vi "Keithley2400_SR830_LakeShore336_4Probe_Resistance_Measurement.vi"() -> ()   [LabVIEW 2018]
uses:
  <instrlib>/Lake Shore 336/Public/Data/Sensor Data (Single Reading).vi
  <instrlib>/Stanford Research 830/Public/Data/Read (All Parameters).vi
  <instrlib>/Keithley 24XX/Public/Data/Read (Single Point).vi
  <instrlib>/Keithley 24XX/Keithley 24XX.lvlib
  <instrlib>/Stanford Research 830/Stanford Research 830.lvlib
  <instrlib>/Lake Shore 336/Lake Shore 336.lvlib
panel:
  out "Gate\nVoltage":sgl
  out "Status":sgl
  out "Leakage \nCurrent":sgl
  in  "Temp Vs Time":enum32{"XY Graph", "Waveform (Time)"}(tab)
  out "Temp vs Time : XYGraph":cluster{"Y":dbl[], "Y":dbl[]}[](graph)
  out "Temp vs Time : TimeGraph":cluster{i32, "Sensor Data":dbl}[](graph)
  in  "Data Source (0:Kelvin)":u16(ring) items=["Kelvin", "Celsius", "Sensor Units"]
  in  "Input (0:A)":u16(ring) items=["A", "B", "C", "D"]
  in  "Serial Configuration 2":T1={"Baud Rate"=57600, "Parity"=1, "Data Bits"=7, "Stop Bits"=10, "Flow Control"=0} {"Flow Control" items=["None", "XON/XOFF", "RTS/CTS", "XON/XOFF & RTS/CTS", "DTR/DSR", "XON/XOFF & DTR/DSR"]; "Stop Bits" items=["1.0"=10, "1.5"=15, "2.0"=20]; "Data Bits" items=["7"=7, "8"=8]; "Parity" items=["None", "Odd", "Even", "Mark", "Space"]; "Baud Rate" items=["300"=300, "600"=600, "1200"=1200, "2400"=2400, "4800"=4800, "9600"=9600, "19200"=19200, "38400"=38400, "57600"=57600]}
  in  "LakeShore 336 esource name":refnum<visa-resource-name>="GPIB0::12::INSTR"
  out "dup path":path
  in  "<File Name>.txt (Don't add extension)":string
  in  "Data Save Path:":path=path "C:/Users/labpc/Documents/ProbeStation Users Data"
  in  "I_leak vs Vg":enum32{"XY Graph", "Waveform (Time)"}(tab)
  out "I_leak vs Vg : XYGraph":cluster{"Y":dbl[], "Y":dbl[]}[](graph)
  out "I_leak vs Vg : TimeGraph":cluster{dbl, "Current":sgl}[](graph)
  in  "Gate Voltage\nInitial (V)":dbl
  out "Gate Voltage\nTraversal Direction":enum16{"Upward", "Downward"}(ring)
  in  "Series Resistance \n(Apparatus Constant)":dbl=10000000.0
  in  "stop":bool
  out "Max/Min(-) \nGate Voltage (V)":dbl=80.0
  in  "Gate Voltage \nStep Size (V)":dbl=0.1
  in  "High Gate \nVoltage (V)":dbl
  in  "Low Gate \nVoltage (V)":dbl
  out "Compliance\n Level (A)":dbl=0.1
  in  "Theta vs Vg":enum32{"XY Graph", "Waveform (Time)"}(tab)
  out "Theta vs Vg : XYGraph":cluster{"Y":dbl[], "Y":dbl[]}[](graph)
  out "Theta vs Vg : TimeGraph":cluster{dbl, "Theta-Value":dbl}[](graph)
  in  "R vs Vg":enum32{"XY Graph", "Waveform (Time)"}(tab)
  out "Resistance vs Vg : XYGraph":cluster{"Y":dbl[], "Y":dbl[]}[](graph)
  out "R vs Vg : TimeGraph":cluster{dbl, dbl}[](graph)
  in  "Sensitivity (Initial Value)":i16(ring)=17 items=["Auto Gain"=-1, "2 nV/fA"=0, "5 nV/fA"=1, "10 nV/fA"=2, "20 nV/fA"=3, "50 nV/fA"=4, "100 nV/fA"=5, "200 nV/fA"=6, "500 nV/fA"=7, "1 uV/pA"=8, "2 uV/pA"=9, "5 uV/pA"=10, "10 uV/pA"=11, "20 uV/pA"=12, "50 uV/pA"=13, "100 uV/pA"=14, "200 uV/pA"=15, "500 uV/pA"=16, "1 mV/nA"=17, "2 mV/nA"=18, "5 mV/nA"=19, "10 mV/nA"=20, "20 mV/nA"=21, "50 mV/nA"=22, "100 mV/nA"=23, "200 mV/nA"=24, "500 mV/mA"=25, "1 V/uA"=26]
  in  "Dynamic Reserve (-1 = Auto)":i16(ring)=-1 items=["Auto Reserve"=-1, "High Reserve"=0, "Normal"=1, "Low Noise"=2]
  in  "Input Connection (0: Single-Ended Voltage)":u16(ring)=1 items=["Single-Ended Voltage", "Differential Voltage", "1 MOhm Current Gain", "100 MOhm Current Gain"]
  out "Input Coupling (0: AC)":u16(ring) items=["AC", "DC"]
  in  "Time Constant (8: 100ms)":u16(ring)=9 items=["10 us", "30 us", "100 us", "300 us", "1 ms", "3 ms", "10 ms", "30 ms", "100 ms", "300 ms", "1 s", "3 s", "10 s", "30 s", "100 s", "300 s", "1 ks", "3 ks", "10 ks", "30 ks"]
  in  "SR830 VISA resource name":refnum<visa-resource-name>="GPIB0::10::INSTR"
  in  "Trigger Source (0: Internal)":u16(ring) items=["Internal", "External"]
  out "Manual Phase (0 Degree)":dbl
  out "Detection Harmonic Number":dbl=1.0
  out "External Reference Trigger (0: Sine Zero Crossing)":u16(ring) items=["Sine Zero Crossing", "TTL Rising Edge", "TTL Falling Edge"]
  in  "Internal Reference Frequency (1000 Hz)":dbl=17.0
  in  "Reference Source (1: Internal)":u16(ring)=1 items=["External", "Internal"]
  in  "Sine Output Amplitude (V)":dbl=1.0
  in  "Serial Configuration":T1={"Baud Rate"=9600, "Parity"=0, "Data Bits"=8, "Stop Bits"=10, "Flow Control"=0} {"Flow Control" items=["None", "XON/XOFF", "RTS/CTS", "XON/XOFF & RTS/CTS", "DTR/DSR", "XON/XOFF & DTR/DSR"]; "Stop Bits" items=["1.0"=10, "1.5"=15, "2.0"=20]; "Data Bits" items=["7"=7, "8"=8]; "Parity" items=["None", "Odd", "Even", "Mark", "Space"]; "Baud Rate" items=["300"=300, "600"=600, "1200"=1200, "2400"=2400, "4800"=4800, "9600"=9600, "19200"=19200]}
  in  "Keithley24XX VISA resource name":refnum<visa-resource-name>="GPIB0::21::INSTR" caption="Keithley 24XX VISA resource name"
  out "Interal Measurement Time":u32
  # "Lake Shore 336 Temp Contr."
  # "SR830 Lock In Amplifier"
  # "MAKE SURE THE SOURCE METER IS ON TO ENSURE NO UNINTENDED JUMPS. PROGRAM WILL KEEP SOURCE METER ON ONCE RUN."
  # "Keithley 2400 SourceMeter"
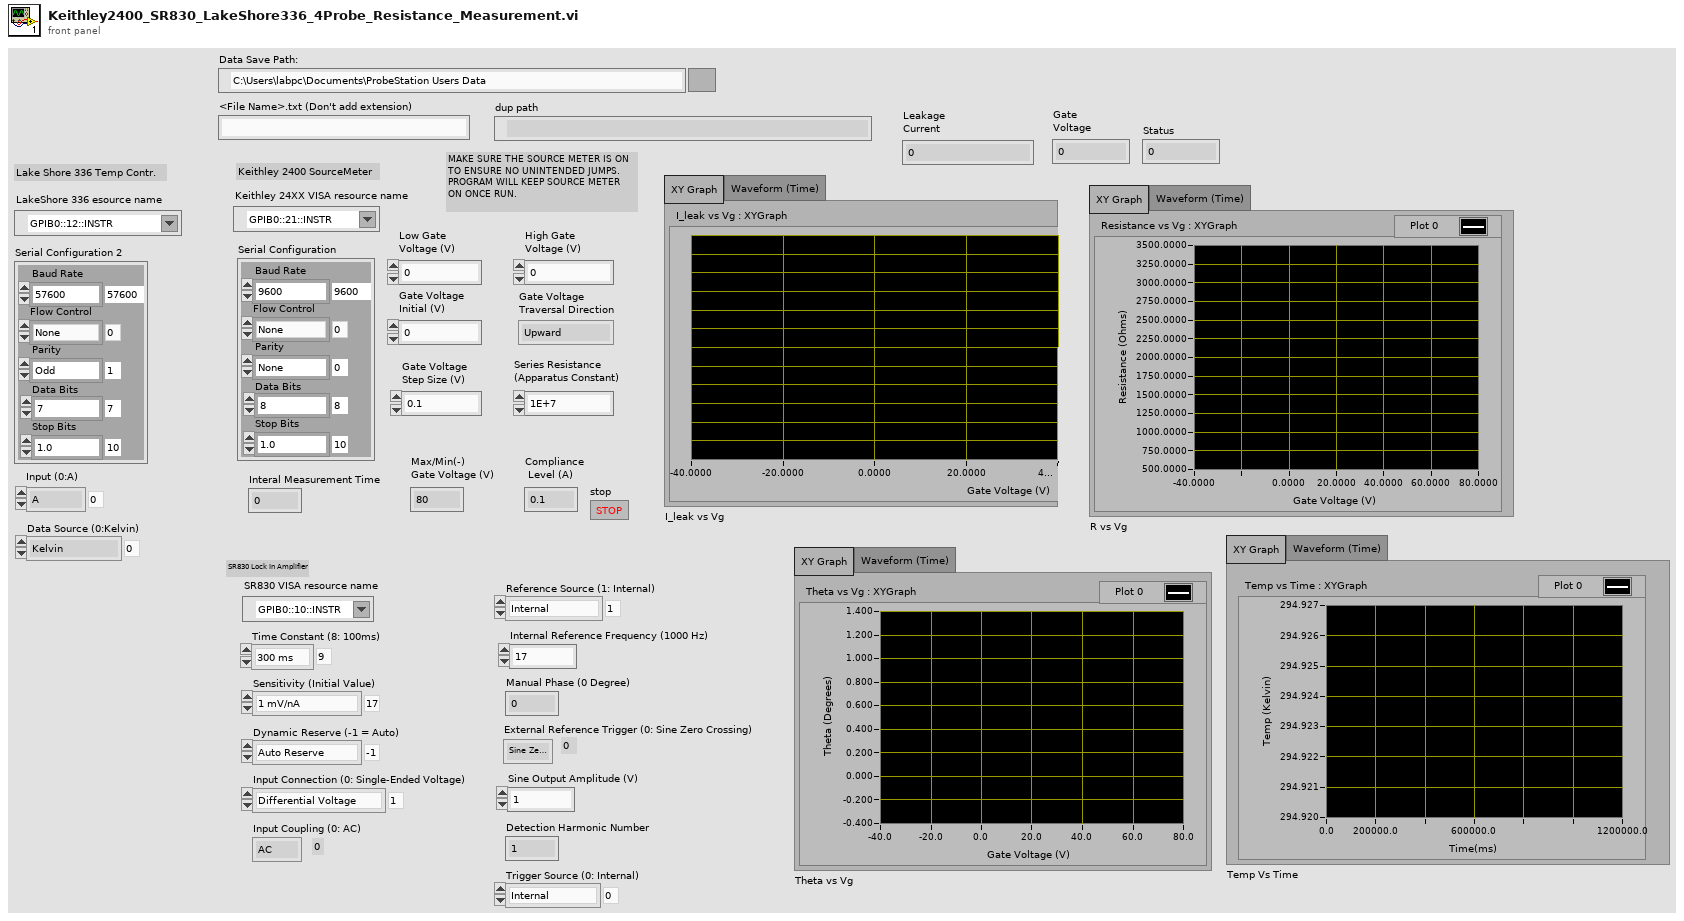
[diagram p1: front panel]
types:
  T1 = cluster{"Baud Rate":u32, "Parity":u16, "Data Bits":u16, "Stop Bits":u16, "Flow Control":u16}
  T2 = enum16{"open", "replace", "create", "open or create", "replace or create", "replace or create with confirmation"}
  T3 = cluster{"X-Value":dbl, "Y-Value":dbl, "R-Value":dbl, "Theta-Value":dbl, "Aux In 1 Value":dbl, "Aux In 2 Value":dbl, "Aux In 3 Value":dbl, "Aux In 4 Value":dbl, "Reference Frequency":dbl, "Channel 1 Display":dbl, "Channel 2 Display":dbl}
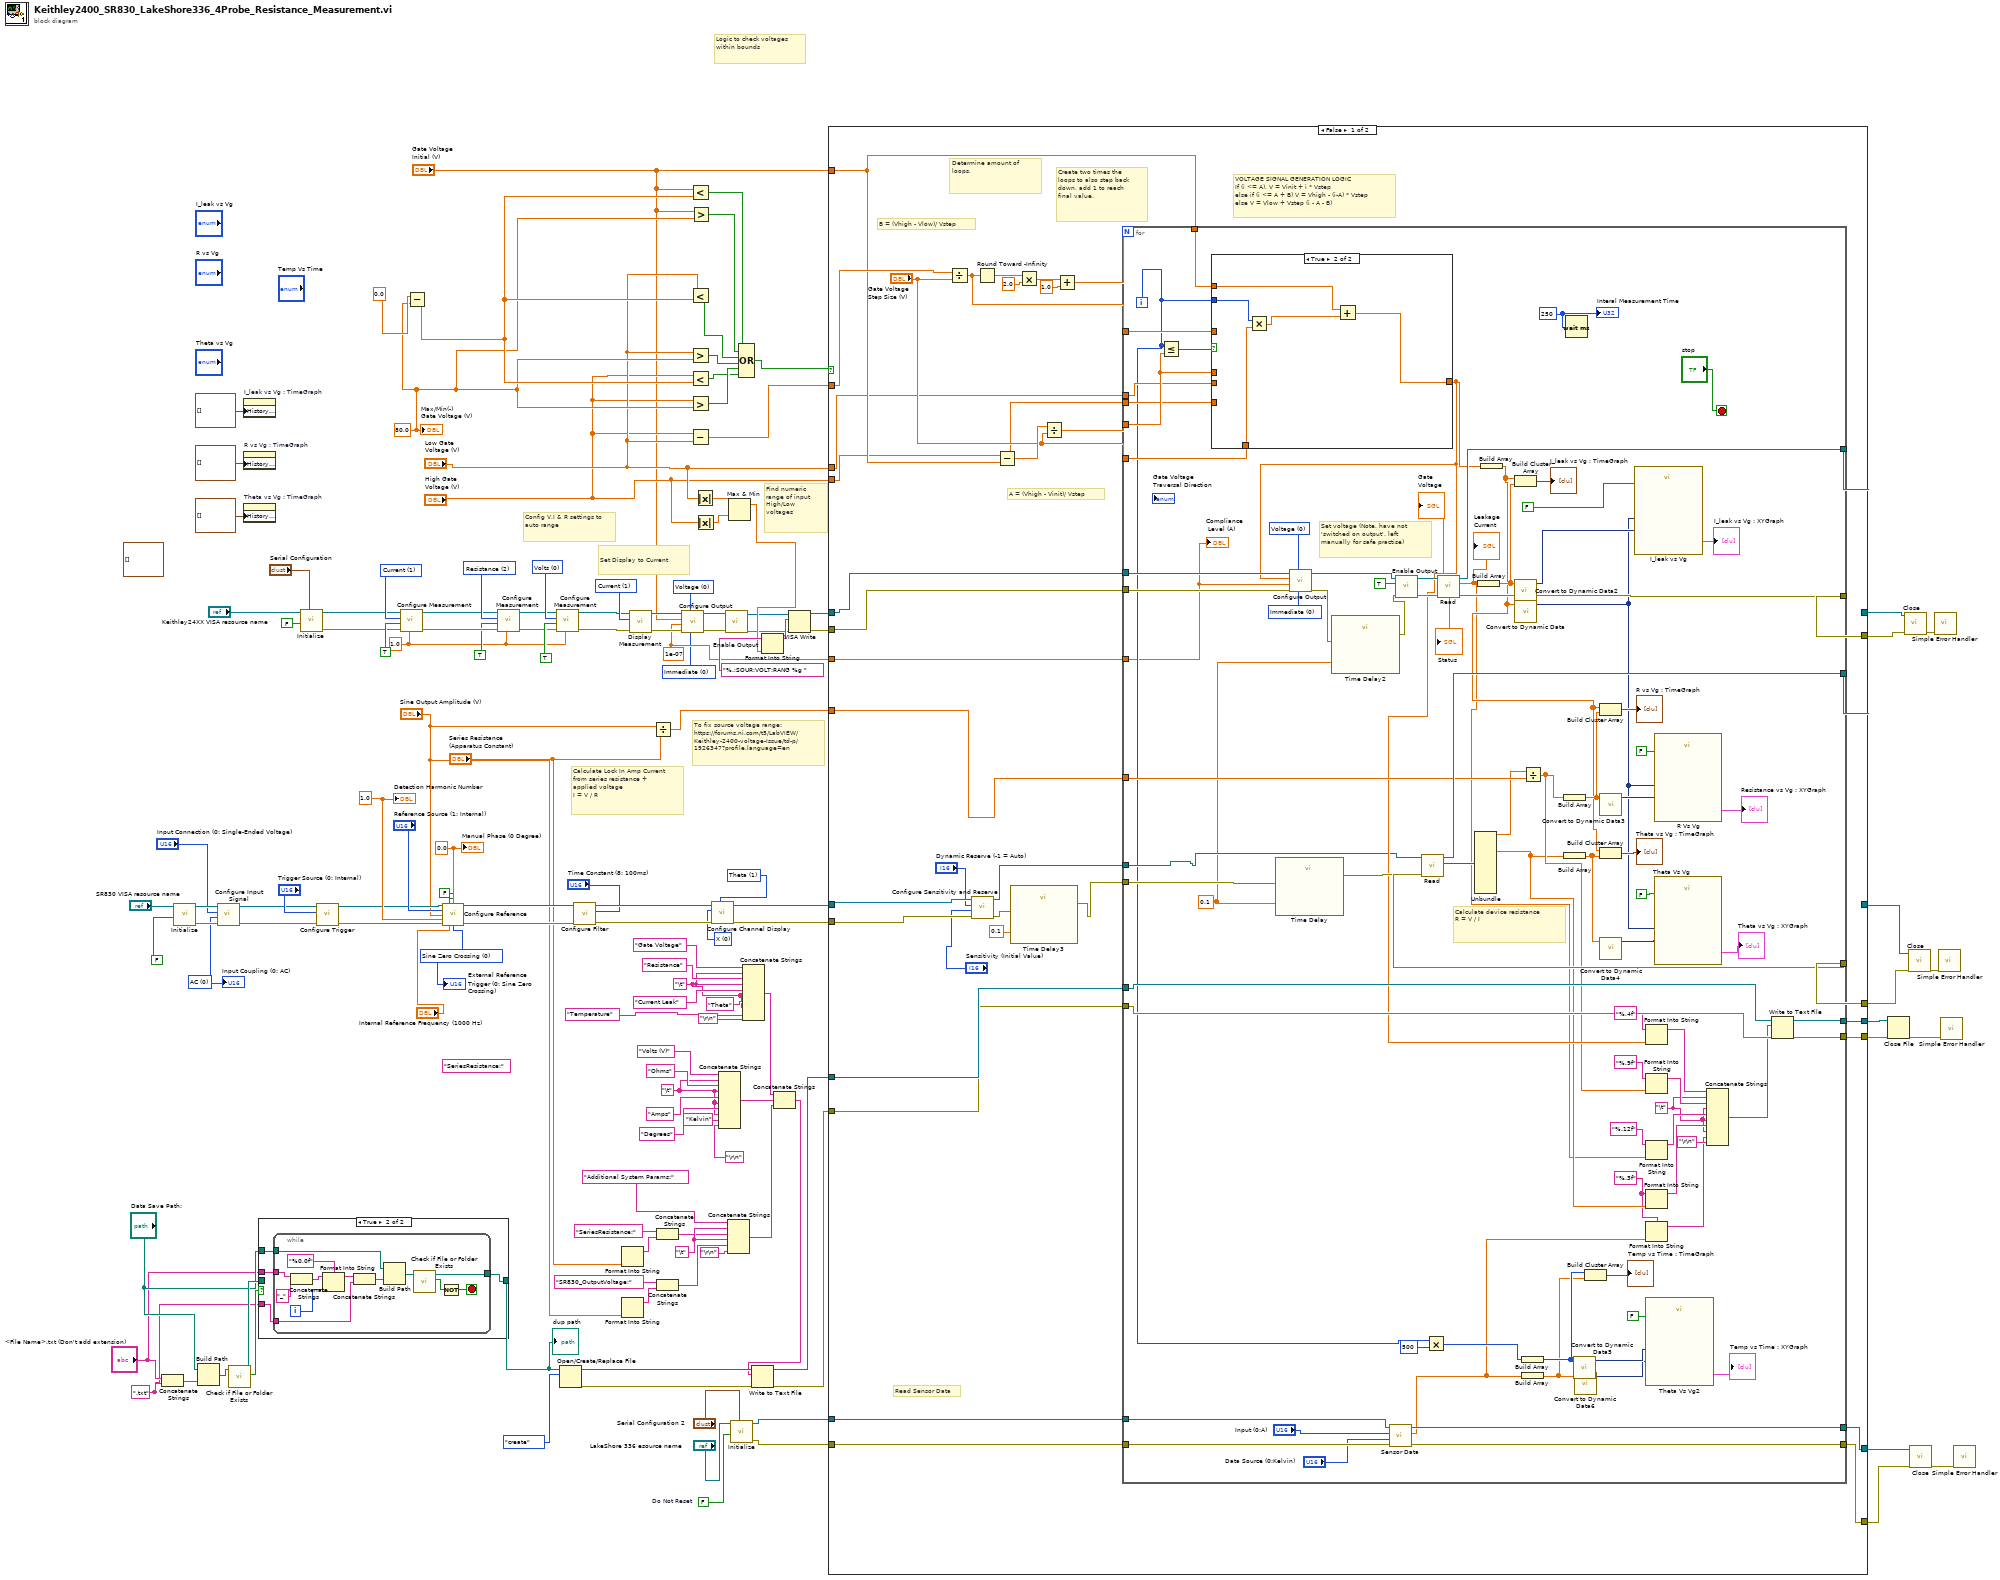
[diagram p0: block diagram]
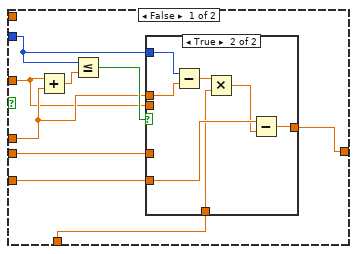
[diagram p3: hidden frame]
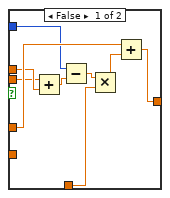
[diagram p4: hidden frame]
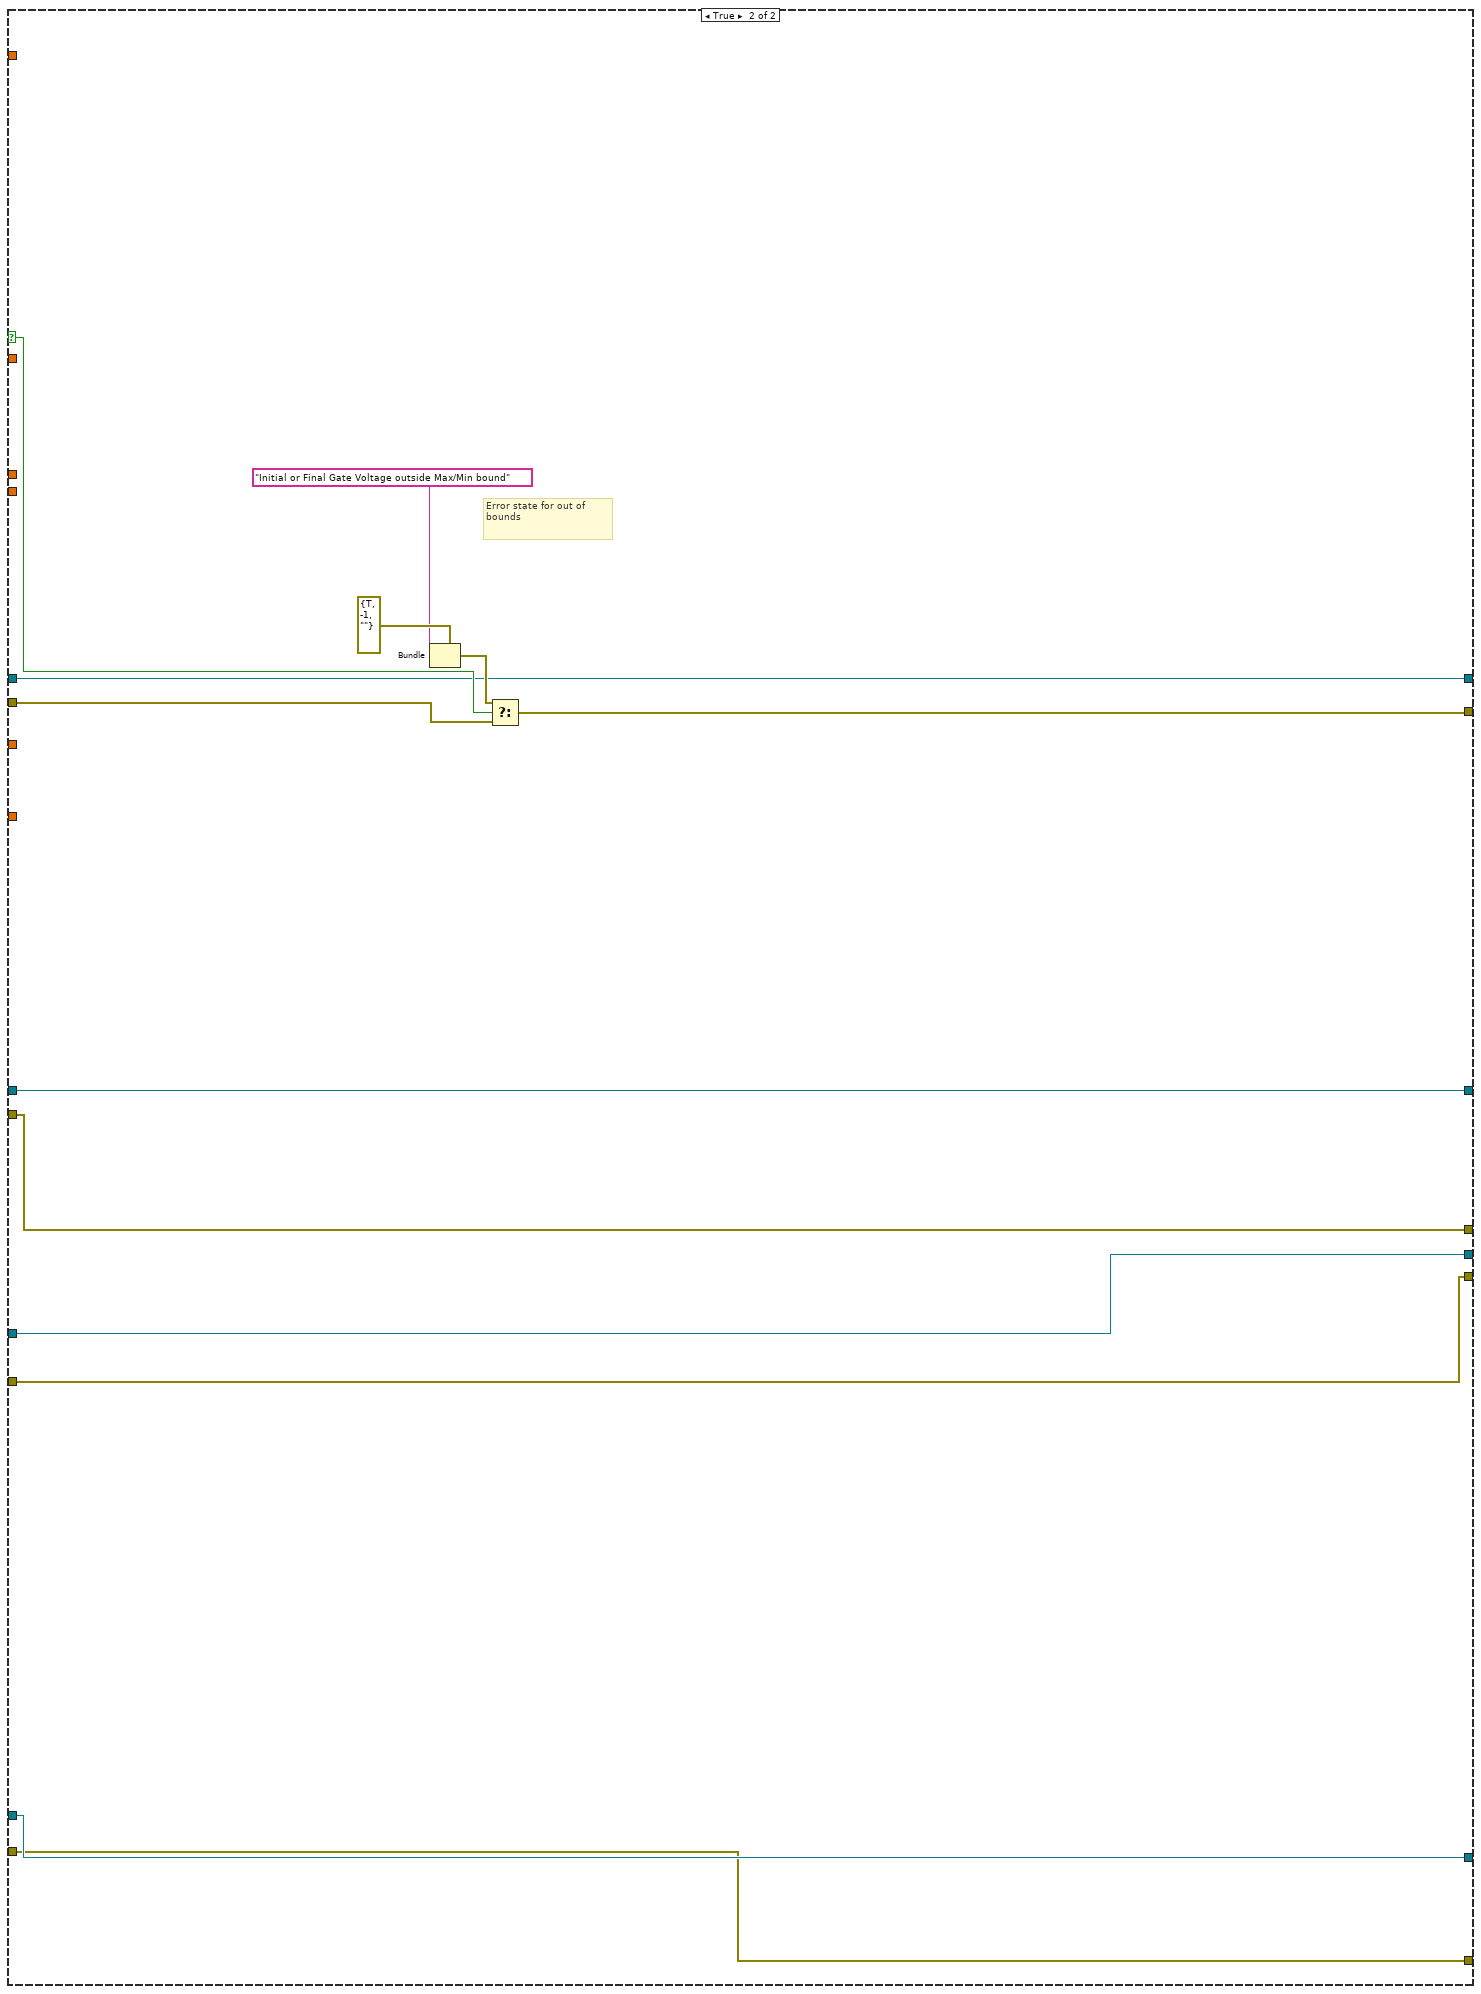
[diagram p5: hidden frame]
diagram:
  w1 = u16 0 items=["Immediate", "Triggered"] ("Output Type  (0: Immediate)")
  w2 = 1e-07 ("Compliance  Level (0.1)")
  w8 = u16 0 items=["Voltage", "Current"] ("Source Mode  (0: Voltage)")
  (unwired) cluster{dbl, "Theta-Value":dbl}[] [] ("History Data")
  w32 = FALSE  # Do Not Reset
  w38 = "\t"
  w21 = "\t"
  w23 = "\t"
  (unwired) "SeriesResistance:" ("string")
  w66 = ".txt"
  w73 = 1.0 ("Manual Range (1.0)")
  w97 = 0.0 ("Manual Phase (0 Degree)")
  w98 = 1.0 ("Detection Harmonic Number (1)")
  w99 = u16 0 items=["Sine Zero Crossing", "TTL Rising Edge", "TTL Falling Edge"] ("External Reference Trigger (0: Sine Zero Crossing)")
  w103 = u16 0 items=["AC", "DC"] ("Input Coupling (0: AC)")
  w85 = u16 0 items=["X", "R", "X Noise", "Aux In 1", "Aux In 2"] ("Channel 1 Display (0: X)")
  w113 = u16 1 items=["Y", "Theta", "Y Noise", "Aux In 3", "Aux In 4"] ("Channel 2 Display  (0: Y)")
  w118 = u16 1 items=["Voltage", "Current", "Resistance"] ("Displayed Measurement (0: Voltage)")
  w127 = u16 2 items=["Volts", "Current", "Resistance"] ("Function (0: Volts)")
  w131 = u16 1 items=["Volts", "Current", "Resistance"] ("Function (0: Volts)")
  w74 = 80.0
  w137 = u16 0 items=["Volts", "Current", "Resistance"] ("Function (0: Volts)")
  # "Find numeric range of input High/Low voltages"
  # "To fix source voltage range:\nhttps://forums.ni.com/t5/LabVIEW/Keithley-2400-voltage-Issue/td-p/1926347?profile.language=en"
  # "Logic to check voltages within bounds"
  # "Calculate Lock In Amp Current from series resistance + applied voltage\nI = V / R"
  # "Set Display to Current"
  # "Config V,I & R settings to auto range"
  n1 = Concatenate Strings("<File Name>.txt (Don't add extension)", w66) -> (w72:string)
  n2 = call <instrlib>:"Initialize.vi"("Reset (True)"=FALSE, "VISA resource name"="SR830 VISA resource name") -> ("error out"=w110:errorcluster, "VISA resource name out"=w111:refnum<visa-resource-name>)  [unwired: 8 in]
  n3 = Build Path(base path="Data Save Path:", name or relative path=w72) -> (appended path=w71:path)
  n4 = call <instrlib>:"Configure Input Signal.vi"("error in (no error)"=w110, "Input Coupling (0: AC)"=w103, "Input Connection (0: Single-Ended Voltage)"="Input Connection (0: Single-Ended Voltage)", "VISA resource name"=w111) -> ("error out"=w94:errorcluster, "VISA resource name out"=w95:refnum<visa-resource-name>)  [unwired: 6 in]
  n5 = call <vilib>:"Check if File or Folder Exists.vi"("path"=w71) -> ("file or folder exists?"=w70:bool, "dup path"=w69:path)  [unwired: 8 in, 1 out]
  n6 = property on="I_leak vs Vg : TimeGraph" class="WFChart (strict)"("History Data"=cluster{dbl, "Current":sgl}[] []) -> ()  [unwired: 2 in, 2 out]
  n7 = property on="R vs Vg : TimeGraph" class="WFChart (strict)"("History Data"=cluster{dbl, dbl}[] []) -> ()  [unwired: 2 in, 2 out]
  n8 = property on="Theta vs Vg : TimeGraph" class="WFChart (strict)"("History Data"=cluster{dbl, "Theta-Value":dbl}[] []) -> ()  [unwired: 2 in, 2 out]
  n9 = case shown="True" w70 {
    tunnel: [w139 w140] -> w63
    tunnel: w69 -> [w139 _]
    tunnel: "Data Save Path:" -> [_ w141]
    tunnel: "<File Name>.txt (Don't add extension)" -> [_ w143]
    tunnel: w66 -> [_ w142]
    frame False {
    }
    frame True {
      n10 = while {
        tunnel: w143 -> [w146]
        tunnel: w142 -> [w151]
        tunnel: w141 -> [w149]
        tunnel: [w147] -> w140
        i -> [w153]
        stop <- w155 stop-if-true
        n11 = Concatenate Strings(w146, "_" ("string")) -> (w145:string)
        n12 = Format Into String(format string="%0.0f", initial string=w145, w153) -> (resulting string=w152:string)  [unwired: 1 in, 1 out]
        n13 = Concatenate Strings(w152, w151) -> (w150:string)
        n14 = Build Path(base path=w149, name or relative path=w150) -> (appended path=w148:path)
        n15 = call <vilib>:"Check if File or Folder Exists.vi"("path"=w148) -> ("file or folder exists?"=w156:bool, "dup path"=w147:path)  [unwired: 8 in, 1 out]
        n16 = Not(x=w156) -> (.not. x?=w155:bool)
      }
    }
  }
  "dup path" <- w63
  n17 = call <instrlib>:"Initialize.vi"("Serial Configuration"="Serial Configuration", "Reset (True)"=FALSE, "VISA resource name"="Keithley24XX VISA resource name") -> ("error out"=w122:errorcluster, "VISA resource name out"=w123:refnum<visa-resource-name>)  [unwired: 7 in]
  n18 = call <instrlib>:"Configure Trigger.vi"("error in (no error)"=w94, "Trigger Source (0: Internal)"="Trigger Source (0: Internal)", "VISA resource name"=w95) -> ("error out"=w92:errorcluster, "VISA resource name out"=w93:refnum<visa-resource-name>)  [unwired: 7 in]
  n19 = call <instrlib>:"Configure Measurement.vi"("Manual Range (1.0)"=w73, "error in (no error)"=w122, "Enable Auto Range (T:Enable)"=TRUE, "Function (0: Volts)"=w131, "VISA resource name"=w123) -> ("error out"=w129:errorcluster, "VISA resource name out"=w124:refnum<visa-resource-name>)  [unwired: 5 in]
  n20 = Subtract(x=0.0, y=w74) -> (x-y=w79:dbl)
  n21 = call <instrlib>:"Configure Reference.vi"("VISA resource name"=w93, "Auto Phase (T: Enabled)"=FALSE, "Manual Phase (0 Degree)"=w97, "Reference Source (1: Internal)"="Reference Source (1: Internal)", "Sine Output Amplitude (1 V)"="Sine Output Amplitude (V)", "Detection Harmonic Number (1)"=w98, "error in (no error)"=w92, "Internal Reference Frequency (1000 Hz)"="Internal Reference Frequency (1000 Hz)", "External Reference Trigger (0: Sine Zero Crossing)"=w99) -> ("VISA resource name out"=w100:refnum<visa-resource-name>, "error out"=w101:errorcluster)  [unwired: 5 in]
  n22 = call <instrlib>:"Configure Measurement.vi"("Manual Range (1.0)"=w73, "error in (no error)"=w129, "Enable Auto Range (T:Enable)"=TRUE, "Function (0: Volts)"=w127, "VISA resource name"=w124) -> ("error out"=w126:errorcluster, "VISA resource name out"=w125:refnum<visa-resource-name>)  [unwired: 5 in]
  n23 = call <instrlib>:"Configure Measurement.vi"("Manual Range (1.0)"=w73, "error in (no error)"=w126, "Enable Auto Range (T:Enable)"=TRUE, "Function (0: Volts)"=w137, "VISA resource name"=w125) -> ("error out"=w116:errorcluster, "VISA resource name out"=w117:refnum<visa-resource-name>)  [unwired: 5 in]
  n24 = Open/Create/Replace File(file path (use dialog)=w63, operation (0:open)=T2."create") -> (refnum out=w64:refnum<file>, error out=w62:errorcluster)  [unwired: 4 in, 1 out]
  n25 = call <instrlib>:"Configure Filter.vi"("error in (no error)"=w101, "Time Constant (8: 100ms)"="Time Constant (8: 100ms)", "VISA resource name"=w100) -> ("error out"=w120:errorcluster, "VISA resource name out"=w119:refnum<visa-resource-name>)  [unwired: 7 in]
  n26 = Format Into String("Series Resistance \n(Apparatus Constant)") -> (resulting string=w56:string)  [unwired: 3 in, 1 out]
  n27 = Format Into String("Sine Output Amplitude (V)") -> (resulting string=w55:string)  [unwired: 3 in, 1 out]
  n28 = call <instrlib>:"Display Measurement.vi"("error in (no error)"=w116, "Displayed Measurement (0: Voltage)"=w118, "VISA resource name"=w117) -> ("error out"=w6:errorcluster, "VISA resource name out"=w7:refnum<visa-resource-name>)  [unwired: 7 in]
  n29 = Divide(x="Sine Output Amplitude (V)", y="Series Resistance \n(Apparatus Constant)") -> (x/y=w91:dbl)
  n30 = Concatenate Strings("SeriesResistance:" ("string"), w56) -> (w37:string)
  n31 = Concatenate Strings("SR830_OutputVoltage:" ("string"), w55) -> (w36:string)
  n32 = call <instrlib>:"Configure Output.vi"("Output Type  (0: Immediate)"=w1, "Source Mode  (0: Voltage)"=w8, "error in (no error)"=w6, "Compliance  Level (0.1)"=w2, "Output Level (0)"="Gate Voltage\nInitial (V)", "VISA resource name"=w7) -> ("error out"=w4:errorcluster, "VISA resource name out"=w5:refnum<visa-resource-name>)  [unwired: 4 in]
  n33 = Less?(x="Gate Voltage\nInitial (V)", y=w79) -> (x < y?=w77:bool)
  n34 = Less?(x="Low Gate \nVoltage (V)", y=w79) -> (x < y?=w83:bool)
  n35 = Greater?(x="Low Gate \nVoltage (V)", y=w74) -> (0:w82:bool)
  n36 = Less?(x="High Gate \nVoltage (V)", y=w79) -> (x < y?=w80:bool)
  n37 = Greater?(x="High Gate \nVoltage (V)", y=w74) -> (0:w81:bool)
  n38 = Subtract(x="High Gate \nVoltage (V)", y="Low Gate \nVoltage (V)") -> (x-y=w75:dbl)
  n39 = Greater?(x="Gate Voltage\nInitial (V)", y=w74) -> (0:w78:bool)
  n40 = Absolute Value(x="Low Gate \nVoltage (V)") -> (abs(x)=w15:dbl)
  n41 = Absolute Value(x="High Gate \nVoltage (V)") -> (abs(x)=w14:dbl)
  n42 = call <instrlib>:"Configure Channel Display.vi"("Channel 2 Display  (0: Y)"=w113, "error in (no error)"=w120, "Channel 1 Display (0: X)"=w85, "VISA resource name"=w119) -> ("error out"=w108:errorcluster, "VISA resource name out"=w109:refnum<visa-resource-name>)  [unwired: 6 in]
  n43 = Concatenate Strings("Volts (V)" ("string"), w21, "Ohms" ("string"), w21, "Amps" ("string"), w21, "Degrees" ("string"), w21, "Kelvin" ("string"), "\r\n") -> (w49:string)
  n44 = call <instrlib>:"Enable Output.vi"("error in (no error)"=w4, "VISA resource name"=w5) -> ("error out"=w9:errorcluster, "VISA resource name out"=w10:refnum<visa-resource-name>)  [unwired: 8 in]
  n45 = Concatenate Strings("Additional System Params:" ("string"), w38, w37, w38, w36, "\r\n") -> (w39:string)
  n46 = Max & Min(x=w15, y=w14) -> (max(x,y)=w13:dbl)  [unwired: 1 out]
  n47 = call <instrlib>:"Initialize.vi"("Serial Configuration"="Serial Configuration 2", "Reset (True)"=w32, "VISA resource name"="LakeShore 336 esource name") -> ("error out"=w27:errorcluster, "VISA resource name out"=w26:refnum<visa-resource-name>)  [unwired: 7 in]
  n48 = Compound Arithmetic op=OR(w77, w78, w83, w82, w81, w80) -> (w76:bool)
  n49 = Concatenate Strings("Gate Voltage" ("string"), w23, "Resistance" ("string"), w23, "Current Leak" ("string"), w23, "Theta" ("string"), w23, "Temperature" ("string"), "\r\n") -> (w50:string)
  n50 = Format Into String(format string="%.;SOUR:VOLT:RANG %g ", w13) -> (resulting string=w19:string)  [unwired: 2 in, 1 out]
  n51 = Concatenate Strings(w50, w49, w39) -> (w34:string)
  n52 = Write to Text File(file (use dialog)=w64, text=w34, error in=w62) -> (refnum out=w60:refnum<file>, error out=w59:errorcluster)  [unwired: 1 in, 1 out]
  n53 = VISA Write(VISA resource name=w10, write buffer=w19, error in (no error)=w9) -> (VISA resource name out=w17:refnum<visa-resource-name>, error out=w16:errorcluster)  [unwired: 1 out]
  n54 = case shown="False" w76 {
    selector: w76 -> [_ w323]
    tunnel: w16 -> [w193 w322]
    tunnel: w17 -> [w158 w317]
    tunnel: [w192 w317] -> w135
    tunnel: [w191 w318] -> w134
    tunnel: w109 -> [w186 w316]
    tunnel: w108 -> [w187 w315]
    tunnel: [w189 w316] -> w107
    tunnel: [w188 w315] -> w106
    tunnel: w91 -> [w183 _]
    tunnel: w75 -> [w178 _]
    tunnel: "Low Gate \nVoltage (V)" -> [w171 _]
    tunnel: "High Gate \nVoltage (V)" -> [w172 _]
    tunnel: "Gate Voltage\nInitial (V)" -> [w174 _]
    tunnel: w60 -> [w167 w314]
    tunnel: w59 -> [w166 w313]
    tunnel: [w165 w314] -> w58
    tunnel: [w164 w313] -> w57
    tunnel: [w160 w311] -> w29
    tunnel: [w159 w312] -> w28
    tunnel: w27 -> [w162 w311]
    tunnel: w26 -> [w161 w312]
    tunnel: w2 -> [w157 _]
    frame False {
      # "Read Sensor Data"
      # "VOLTAGE SIGNAL GENERATION LOGIC\nIf (i <= A), V = Vinit + i * Vstep\nelse if (i <= A + B) V = Vhigh - (i-A) * Vstep\nelse V = Vlow + Vstep (i - A - B)"
      # "B = (Vhigh - Vlow)/ Vstep"
      # "A = (Vhigh - Vinit)/ Vstep"
      # "Create two times the loops to also step back down, add 1 to reach final value."
      # "Determine amount of loops,"
      n55 = Divide(x=w178, y="Gate Voltage \nStep Size (V)") -> (x/y=w173:dbl)
      n56 = call <instrlib>:"Configure Sensitivity and Reserve.vi"("error in (no error)"=w187, "Sensitivity (-1: Auto gain)"="Sensitivity (Initial Value)", "Dynamic Reserve (-1: Auto Reserve)"="Dynamic Reserve (-1 = Auto)", "VISA resource name"=w186) -> ("error out"=w169:errorcluster, "VISA resource name out"=w185:refnum<visa-resource-name>)  [unwired: 6 in]
      n57 = Round Toward -Infinity(1:w173) -> (0:w181:dbl)
      n58 = Subtract(x=w172, y=w174) -> (x-y=w177:dbl)
      n59 = call "Time Delay3"("error in (no error)"=w169, "Delay Time (s)"=0.1) -> ("error out"=w170:errorcluster)  [unwired: 9 in]
      n60 = Multiply(x=w181, y=2.0) -> (x*y=w180:dbl)
      n61 = Divide(x=w177, y="Gate Voltage \nStep Size (V)") -> (x/y=w175:dbl)
      n62 = Add(x=w180, y=1.0) -> (x+y=w179:dbl)
      n63 = for {
        N: w179 -> [_]
        tunnel: w158 -> [w276]
        tunnel: w193 -> [w241]
        tunnel: [w280] -> w192
        tunnel: [w279] -> w191
        tunnel: [w269] -> w189
        tunnel: [w270] -> w188
        tunnel: w185 -> [w222]
        tunnel: w170 -> [w223]
        tunnel: w183 -> [w267]
        tunnel: "Gate Voltage \nStep Size (V)" -> [w247]
        tunnel: w175 -> [w245]
        tunnel: w174 -> [w248]
        tunnel: w173 -> [w246]
        tunnel: w172 -> [w244]
        tunnel: w171 -> [w243]
        tunnel: w167 -> [w238]
        tunnel: w166 -> [w237]
        tunnel: [w236] -> w165
        tunnel: [w235] -> w164
        tunnel: w162 -> [w214]
        tunnel: w161 -> [w213]
        tunnel: [w212] -> w160
        tunnel: [w211] -> w159
        tunnel: w157 -> [w194]
        i -> [w205]
        stop <- "stop" stop-if-true
        w202 = "%.3f" ("format string")
        w199 = "\t"
        w242 = u16 0 items=["Immediate", "Triggered"] ("Output Type  (0: Immediate)")
        w221 = 0.1 ("Delay Time (s)")
        w277 = u32 250 ("milliseconds to wait")
        w272 = u16 0 items=["Voltage", "Current"] ("Source Mode  (0: Voltage)")
        # "Calculate device resistance\nR = V / I"
        # "Set voltage (Note, have not 'switched on output', left manually for safe practise)"
        n64 = Less Or Equal?(x=w205, y=w245) -> (x <= y?=w249:bool)
        n65 = case shown="True" w249 {
          tunnel: [w287 w306] -> w229
          tunnel: w248 -> [_ w309]
          tunnel: w205 -> [w284 w310]
          tunnel: w247 -> [w285 w307]
          tunnel: w246 -> [w281 _]
          tunnel: w245 -> [w283 _]
          tunnel: w244 -> [w286 _]
          tunnel: w243 -> [w282 _]
          frame False {
            n66 = Add(x=w281, y=w283) -> (x+y=w288:dbl)
            n67 = Less Or Equal?(x=w284, y=w288) -> (x <= y?=w289:bool)
            n68 = case shown="True" w289 {
              tunnel: [w295 w304] -> w287
              tunnel: w286 -> [_ w305]
              tunnel: w285 -> [w297 w302]
              tunnel: w284 -> [w292 w301]
              tunnel: w283 -> [w291 w300]
              tunnel: w282 -> [w298 _]
              tunnel: w281 -> [w290 _]
              frame False {
                n69 = Add(x=w290, y=w291) -> (x+y=w293:dbl)
                n70 = Subtract(x=w292, y=w293) -> (x-y=w294:dbl)
                n71 = Multiply(x=w294, y=w297) -> (x*y=w296:dbl)
                n72 = Add(x=w298, y=w296) -> (x+y=w295:dbl)
              }
              frame True {
                n73 = Subtract(x=w301, y=w300) -> (x-y=w303:dbl)
                n74 = Multiply(x=w303, y=w302) -> (x*y=w299:dbl)
                n75 = Subtract(x=w305, y=w299) -> (x-y=w304:dbl)
              }
            }
          }
          frame True {
            n76 = Multiply(x=w310, y=w307) -> (x*y=w308:dbl)
            n77 = Add(x=w309, y=w308) -> (x+y=w306:dbl)
          }
        }
        n78 = call "Time Delay"("error in (no error)"=w223, "Delay Time (s)"=w221) -> ("error out"=w265:errorcluster)  [unwired: 9 in]
        n79 = call <instrlib>:"Configure Output.vi"("Output Type  (0: Immediate)"=w242, "Source Mode  (0: Voltage)"=w272, "error in (no error)"=w241, "Compliance  Level (0.1)"=w194, "Output Level (0)"=w229, "VISA resource name"=w276) -> ("error out"=w240:errorcluster, "VISA resource name out"=w275:refnum<visa-resource-name>)  [unwired: 4 in]
        n80 = call "Time Delay2"("error in (no error)"=w240, "Delay Time (s)"=w221) -> ("error out"=w239:errorcluster)  [unwired: 9 in]
        n81 = call-poly <instrlib>:"Sensor Data.vi"("error in (no error)"=w214, "Data Source (0:Kelvin)"="Data Source (0:Kelvin)", "Input (0:A)"="Input (0:A)", "VISA resource name"=w213) -> ("error out"=w212:errorcluster, "Sensor Data"=w201:dbl, "VISA resource name out"=w211:refnum<visa-resource-name>)  [unwired: 5 in]
        n82 = call <instrlib>:"Enable Output.vi"("error in (no error)"=w239, "Enable Output (T: Enable)"=TRUE, "VISA resource name"=w275) -> ("error out"=w274:errorcluster, "VISA resource name out"=w273:refnum<visa-resource-name>)  [unwired: 7 in]
        n83 = call-poly <instrlib>:"Read.vi"("error in (no error)"=w265, "VISA resource name"=w222) -> ("error out"=w270:errorcluster, "Parameter Values"=w268:T3, "VISA resource name out"=w269:refnum<visa-resource-name>)  [unwired: 7 in]
        n84 = Multiply(x=w205, y=500) -> (x*y=w203:i32)
        n85 = call-poly <instrlib>:"Read.vi"("VISA resource name"=w273, "error in (no error)"=w274) -> ("Voltage"=→"Gate\nVoltage":sgl, "VISA resource name out"=w280:refnum<visa-resource-name>, "Current"=w197:sgl, "Status"=→"Status":sgl, "error out"=w279:errorcluster)  [unwired: 7 in, 2 out]
        "Leakage \nCurrent" <- w197
        n86 = Unbundle(w268) -> ("X-Value"=w266:dbl, "Theta-Value"=w227:dbl)  [unwired: 9 out]
        n87 = Build Array(w197) -> (w262:sgl[])
        n88 = Build Array(w229) -> (w218:dbl[])
        n89 = Build Cluster Array(w218, w262) -> (→"I_leak vs Vg : TimeGraph":cluster{dbl, "Current":sgl}[])
        n90 = call "Convert to Dynamic Data2"("Array"=w262) -> ("Dynamic Data Type"=w261:dynamicdata)  [unwired: 3 in]
        n91 = call "Convert to Dynamic Data"("Array"=w218) -> ("Dynamic Data Type"=w217:dynamicdata)  [unwired: 3 in]
        n92 = Build Array(w203) -> (w215:i32[])
        n93 = Build Array(w201) -> (w207:dbl[])
        n94 = Divide(x=w266, y=w267) -> (x/y=w228:dbl)
        n95 = Build Array(w228) -> (w260:dbl[])
        n96 = Build Array(w227) -> (w258:dbl[])
        n97 = Wait (ms)(milliseconds to wait=w277) -> ()  [unwired: 1 out]
        n98 = call "Convert to Dynamic Data5"("Array"=w215) -> ("Dynamic Data Type"=w216:dynamicdata)  [unwired: 3 in]
        n99 = call "Convert to Dynamic Data6"("Array"=w207) -> ("Dynamic Data Type"=w208:dynamicdata)  [unwired: 3 in]
        n100 = Build Cluster Array(w215, w207) -> (→"Temp vs Time : TimeGraph":cluster{i32, "Sensor Data":dbl}[])
        n101 = Build Cluster Array(w218, w260) -> (→"R vs Vg : TimeGraph":cluster{dbl, dbl}[])
        n102 = call "Convert to Dynamic Data3"("Array"=w260) -> ("Dynamic Data Type"=w259:dynamicdata)  [unwired: 3 in]
        n103 = Build Cluster Array(w218, w258) -> (→"Theta vs Vg : TimeGraph":cluster{dbl, "Theta-Value":dbl}[])
        n104 = call "Convert to Dynamic Data4"("Array"=w258) -> ("Dynamic Data Type"=w257:dynamicdata)  [unwired: 3 in]
        n105 = call "I_leak vs Vg"("Reset"=FALSE, "Y Input"=w261, "X Input"=w217) -> ("XY Graph"=→"I_leak vs Vg : XYGraph":cluster{"X":dbl[], "Y":dbl[]}[])  [unwired: 7 in, 1 out]
        n106 = Format Into String(format string="%.4f", w229) -> (resulting string=w234:string)  [unwired: 2 in, 1 out]
        n107 = Format Into String(format string="%.9f", w228) -> (resulting string=w233:string)  [unwired: 2 in, 1 out]
        n108 = Format Into String(format string="%.12f", w197) -> (resulting string=w232:string)  [unwired: 2 in, 1 out]
        n109 = Format Into String(format string=w202, w227) -> (resulting string=w231:string)  [unwired: 2 in, 1 out]
        n110 = Format Into String(format string=w202, w201) -> (resulting string=w198:string)  [unwired: 2 in, 1 out]
        n111 = call "Theta Vs Vg2"("Reset"=FALSE, "Y Input"=w208, "X Input"=w216) -> ("XY Graph"=→"Temp vs Time : XYGraph":cluster{"X":dbl[], "Y":dbl[]}[])  [unwired: 7 in, 1 out]
        n112 = call "R Vs Vg"("Reset"=FALSE, "Y Input"=w259, "X Input"=w217) -> ("XY Graph"=→"Resistance vs Vg : XYGraph":cluster{"X":dbl[], "Y":dbl[]}[])  [unwired: 7 in, 1 out]
        n113 = call "Theta Vs Vg"("Reset"=FALSE, "Y Input"=w257, "X Input"=w217) -> ("XY Graph"=→"Theta vs Vg : XYGraph":cluster{"X":dbl[], "Y":dbl[]}[])  [unwired: 7 in, 1 out]
        n114 = Concatenate Strings(w234, w199, w233, w199, w232, w199, w231, w199, w198, "\r\n") -> (w230:string)
        n115 = Write to Text File(file (use dialog)=w238, text=w230, error in=w237) -> (refnum out=w236:refnum<file>, error out=w235:errorcluster)  [unwired: 1 in, 1 out]
        "Compliance\n Level (A)" <- w194
        "Interal Measurement Time" <- w277
      }
    }
    frame True {
      # "Error state for out of bounds"
      n116 = Bundle(cluster=errorcluster {"status"=TRUE, "code"=-1, "source"=""} ("error constant"), "source"="Initial or Final Gate Voltage outside Max/Min bound") -> (w319:errorcluster)  [unwired: 2 in]
      n117 = Select(t=w319, s=w323, f=w322) -> (s? t:f=w318:errorcluster)
    }
  }
  n118 = Close File(refnum=w58, error in=w57) -> (error out=w61:errorcluster)  [unwired: 1 out]
  n119 = call <instrlib>:"Close.vi"("error in (no error)"=w134, "VISA resource name"=w135) -> ("error out"=w133:errorcluster)  [unwired: 9 in]
  n120 = call <instrlib>:"Close.vi"("error in (no error)"=w106, "VISA resource name"=w107) -> ("error out"=w121:errorcluster)  [unwired: 9 in]
  n121 = call <instrlib>:"Close.vi"("error in (no error)"=w29, "VISA resource name"=w28) -> ("error out"=w30:errorcluster)  [unwired: 9 in]
  n122 = call <vilib>:"Simple Error Handler.vi"("error in (no error)"=w133) -> ()  [unwired: 4 in, 5 out]
  n123 = call <vilib>:"Simple Error Handler.vi"("error in (no error)"=w121) -> ()  [unwired: 4 in, 5 out]
  n124 = call <vilib>:"Simple Error Handler.vi"("error in (no error)"=w61) -> ()  [unwired: 4 in, 5 out]
  n125 = call <vilib>:"Simple Error Handler.vi"("error in (no error)"=w30) -> ()  [unwired: 4 in, 5 out]
  "Max/Min(-) \nGate Voltage (V)" <- w74
  "Input Coupling (0: AC)" <- w103
  "External Reference Trigger (0: Sine Zero Crossing)" <- w99
  "Detection Harmonic Number" <- w98
  "Manual Phase (0 Degree)" <- w97
